vi "Instrument Setup.vi"(3 "Configured Inst":T1[](array[typedef])=[{"Public"={"Column Name"=["Timestamp"], "Trace Color"=[13802409]}, "Private"={"Path"=path "", "VI Refnum"=refnum, "Name"="", "# of Values"=0, "Scale Factors"=[], "Display"=[], "Offset"=[1.0]}}, {"Public"={"Column Name"=["Timestamp"], "Trace Color"=[11567897]}, "Private"={"Path"=path "", "VI Refnum"=refnum, "Name"="", "# of Values"=0, "Scale Factors"=[], "Display"=[], "Offset"=[1.0]}}, {"Public"={"Column Name"=[], "Trace Color"=[]}, "Private"={"Path"=path "", "VI Refnum"=refnum, "Name"="", "# of Values"=0, "Scale Factors"=[], "Display"=[], "Offset"=[1.0]}}] {"Private"."Offset" format="%^_3e"; "Private"."Scale Factors" format="%^_3e"}) -> (1 "Configured Inst dup":T1[](array[typedef]) {"Private"."Offset" format="%^_3e"; "Private"."Scale Factors" format="%^_3e"})   [LabVIEW 2021]
uses:
  Sub Controls/Instrument Properties.ctl
  Sub Controls/Public.ctl
  Sub Controls/Private.ctl
  Sub Controls/Instrument Ref.ctl
  Sub Controls/SystemCheckBox-resize.ctl
  <vilib>/Utility/miscctls.llb/LVBoundsTypeDef.ctl
  Sub Controls/Instrument Info.ctl
panel:
  out "Scan Indicator":string="Scanning Instruments...."
  in  "Rescan":bool
  in  "Instrument List":i32(listbox)
  in  "Delete":bool
  in  "Insert":bool
  in  "Done":bool
  in  "Configured Instruments":i32(listbox)
  # "Use the buttons or drag and drop instruments from the List to the Configured column.   Arrange configured instruments in the order to be called."
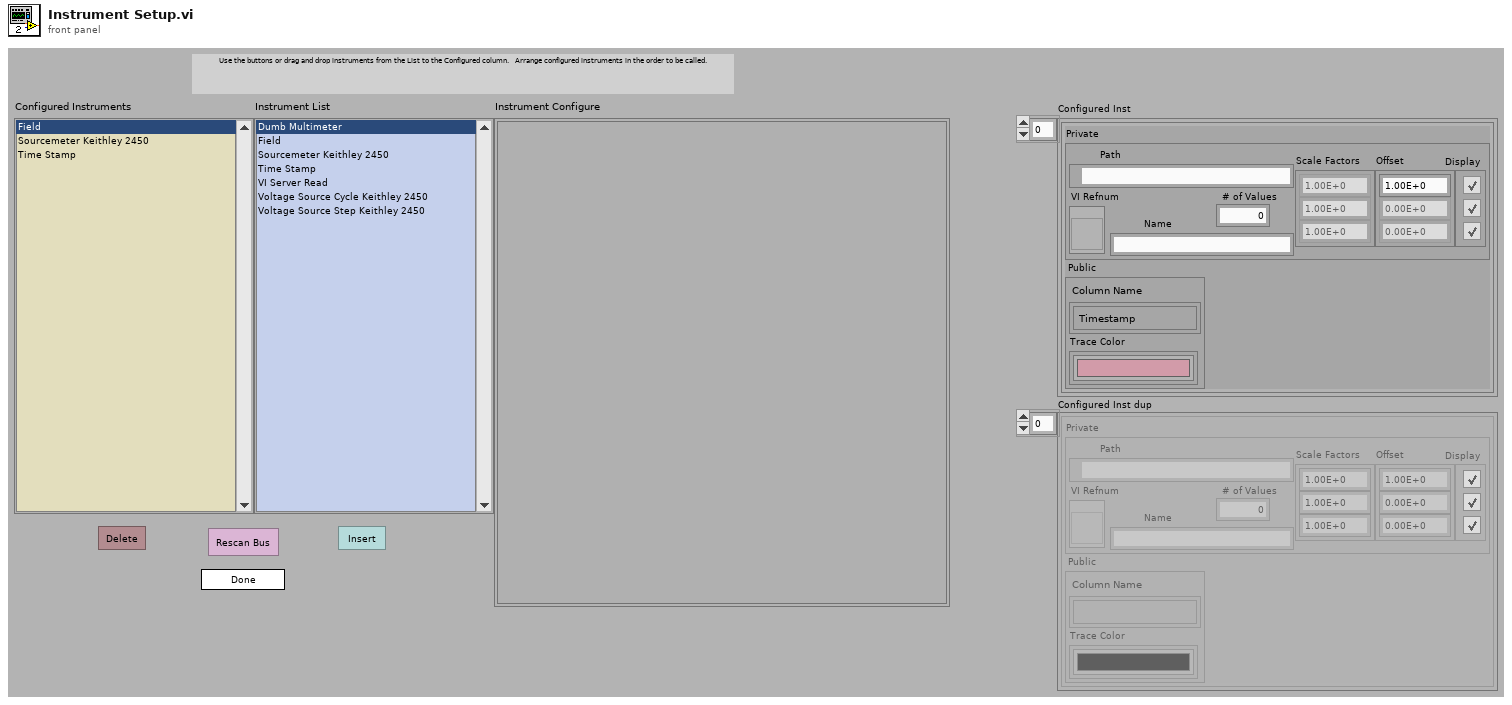
[diagram p1: front panel]
types:
  T1 = typedef "Instrument Properties.ctl" = cluster{"Public":T2, "Private":T3}
  T2 = typedef "Public.ctl" = cluster{"Column Name":string[], "Trace Color":u32[]}
  T3 = typedef "Private.ctl" = cluster{"Path":path, "VI Refnum":T4, "Name":string, "# of Values":i32, "Scale Factors":dbl[], "Display":T5[], "Offset":dbl[]}
  T4 = typedef "Instrument Ref.ctl" = refnum<vi>
  T5 = typedef "SystemCheckBox-resize.ctl" = bool
  T6 = typedef "Instrument Info.ctl" = cluster{"Name":string, "path":path}
  T7 = typedef "LVBoundsTypeDef.ctl" = cluster{"Width":u32, "Height":u32}
  T8 = enum8{"Enabled", "Disabled", "Disabled and Grayed Out"}
  T9 = typedef "Instrument IDN.ctl" = cluster{"VISA Address":string, "Status":u16, "Manufacturer":string, "Model":string, "Info":string, "Info 2":string, "Misc Data":variant}
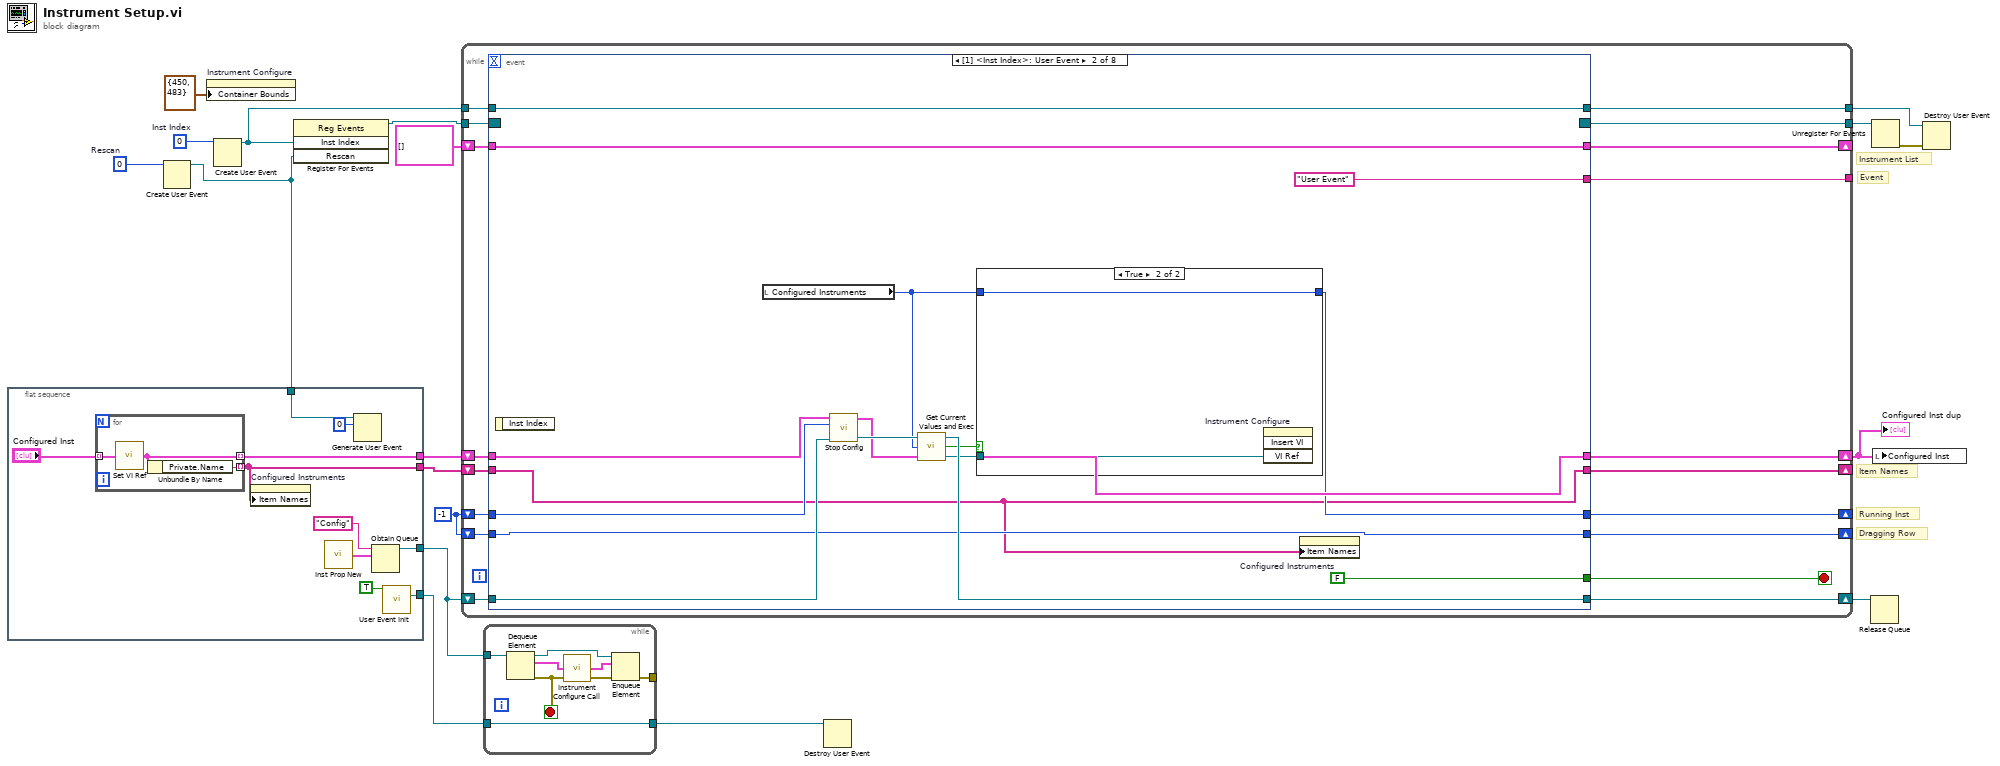
[diagram p0: block diagram]
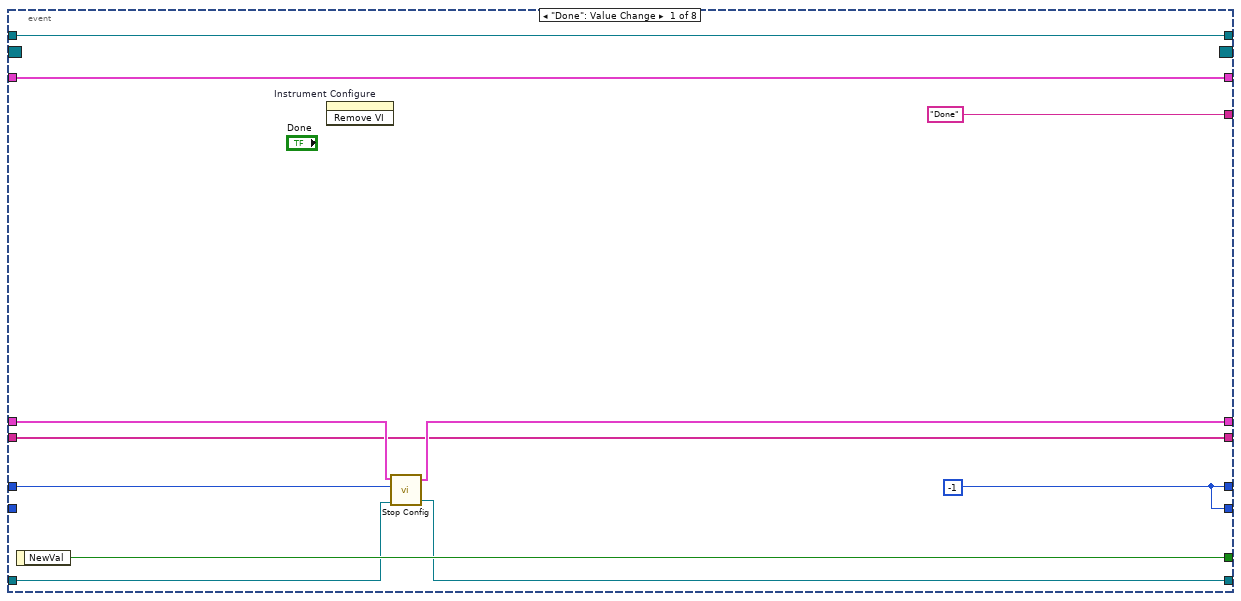
[diagram p2: hidden frame]
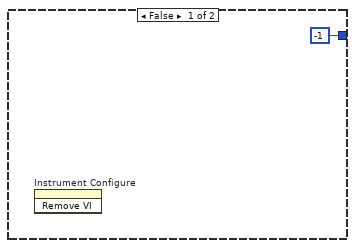
[diagram p3: hidden frame]
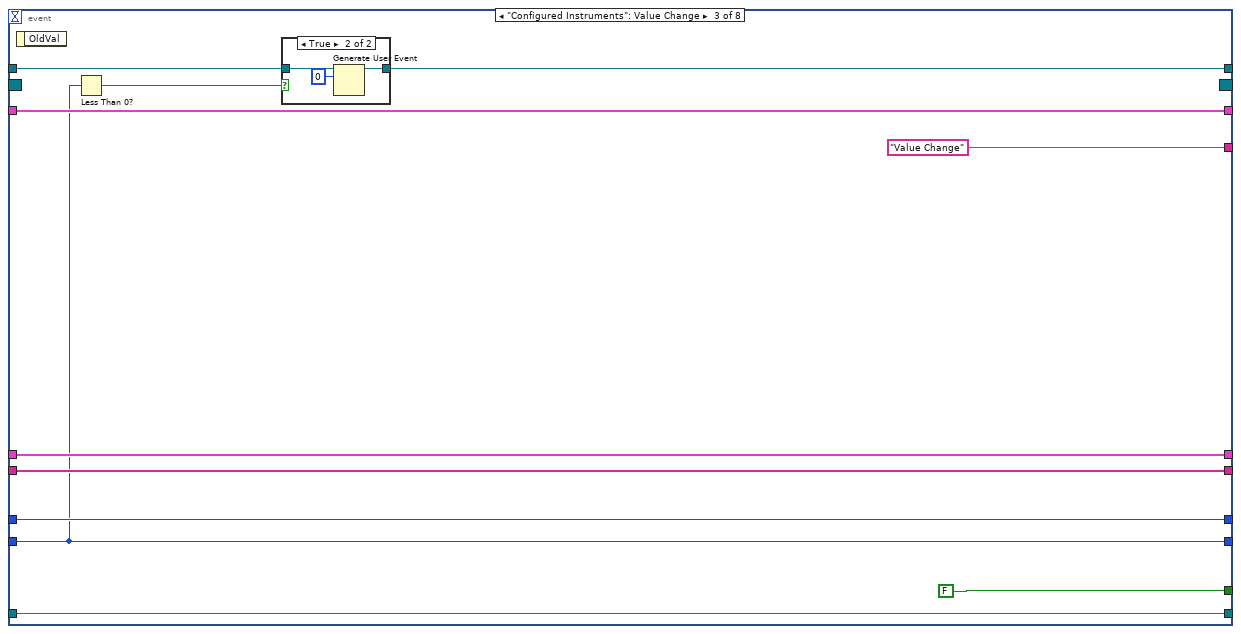
[diagram p4: hidden frame]
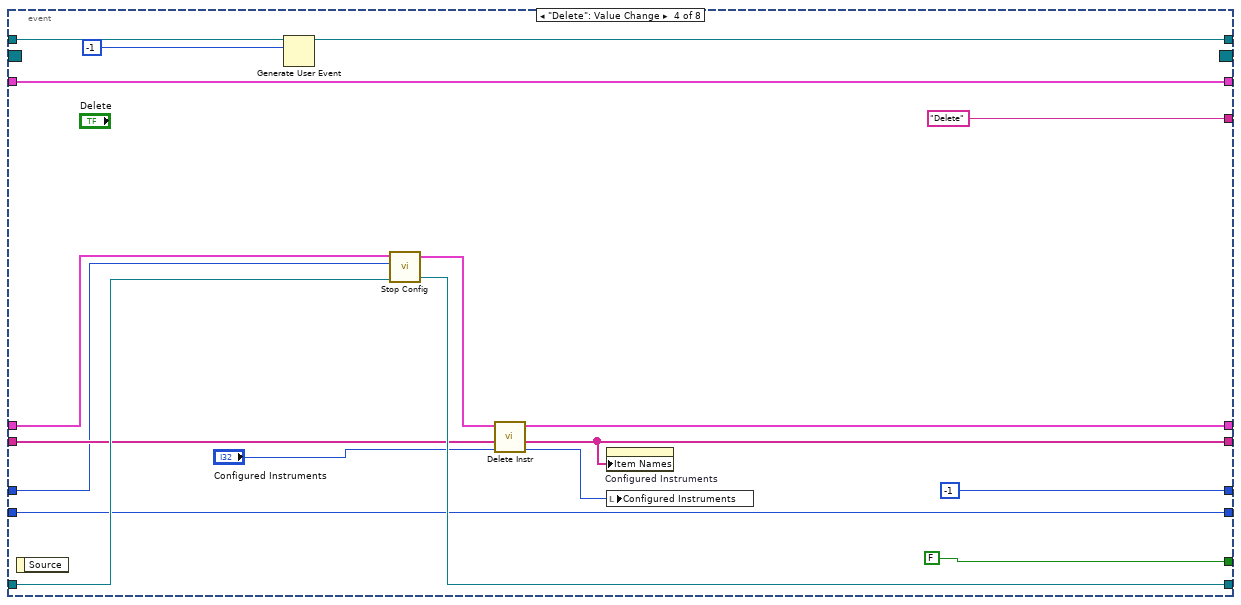
[diagram p6: hidden frame]
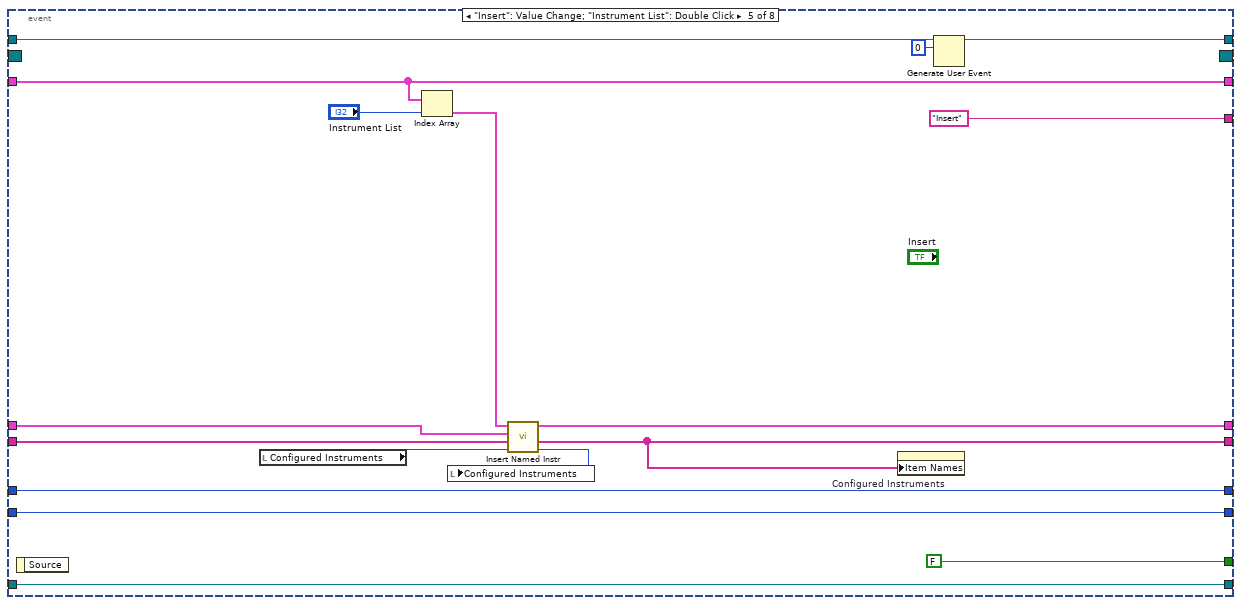
[diagram p7: hidden frame]
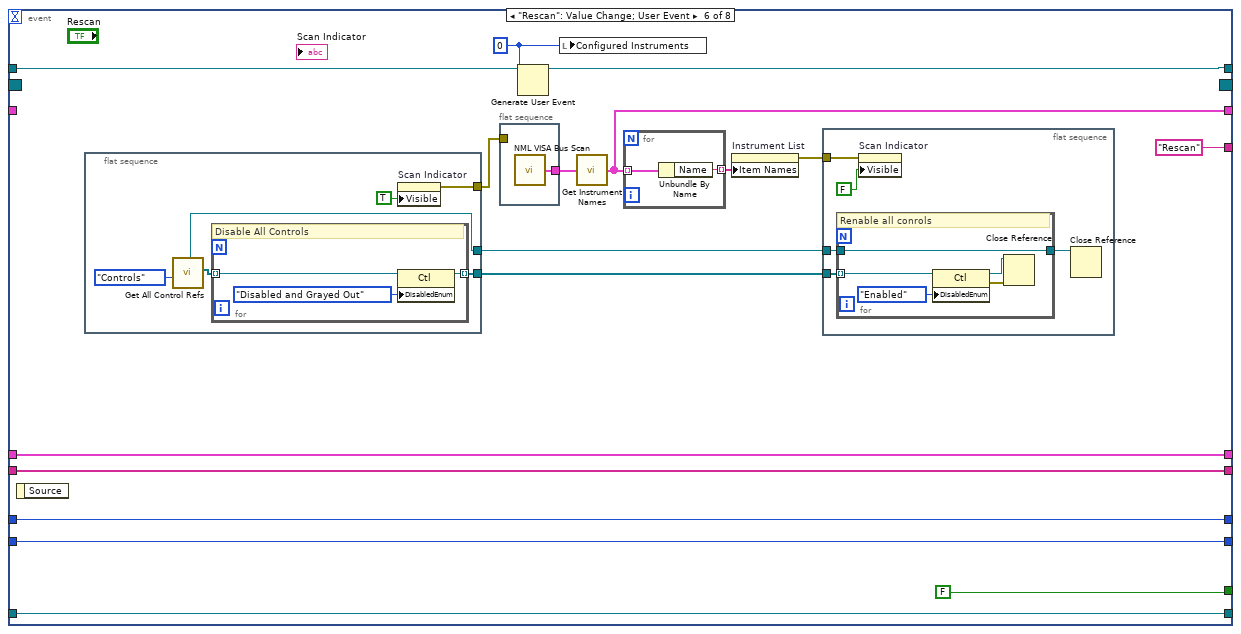
[diagram p8: hidden frame]
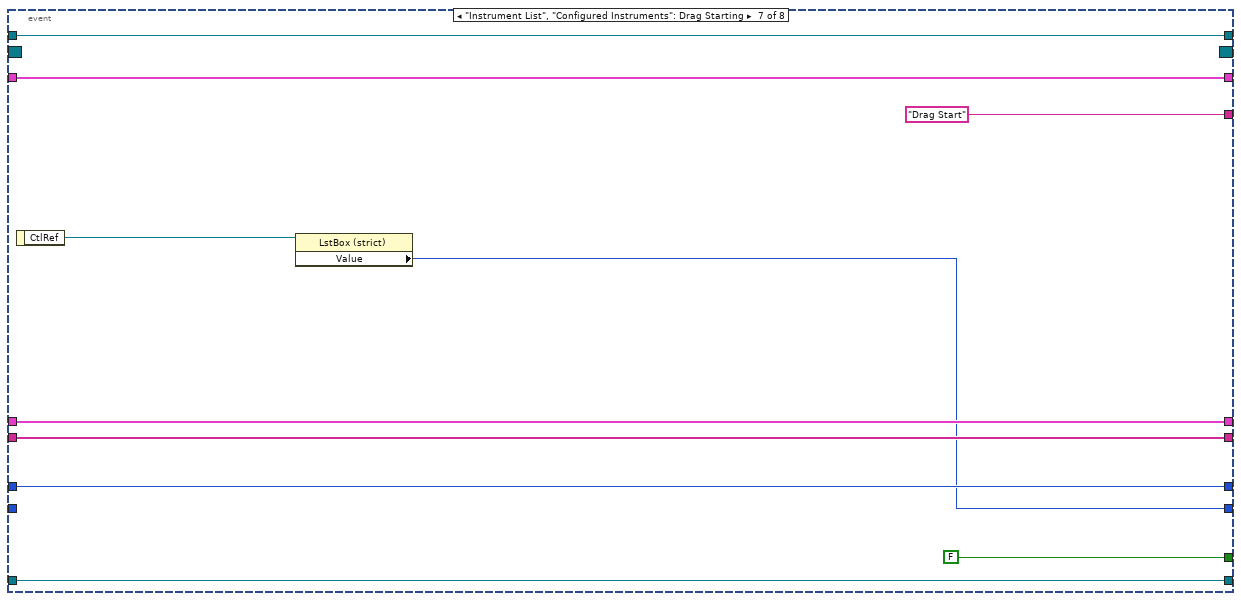
[diagram p9: hidden frame]
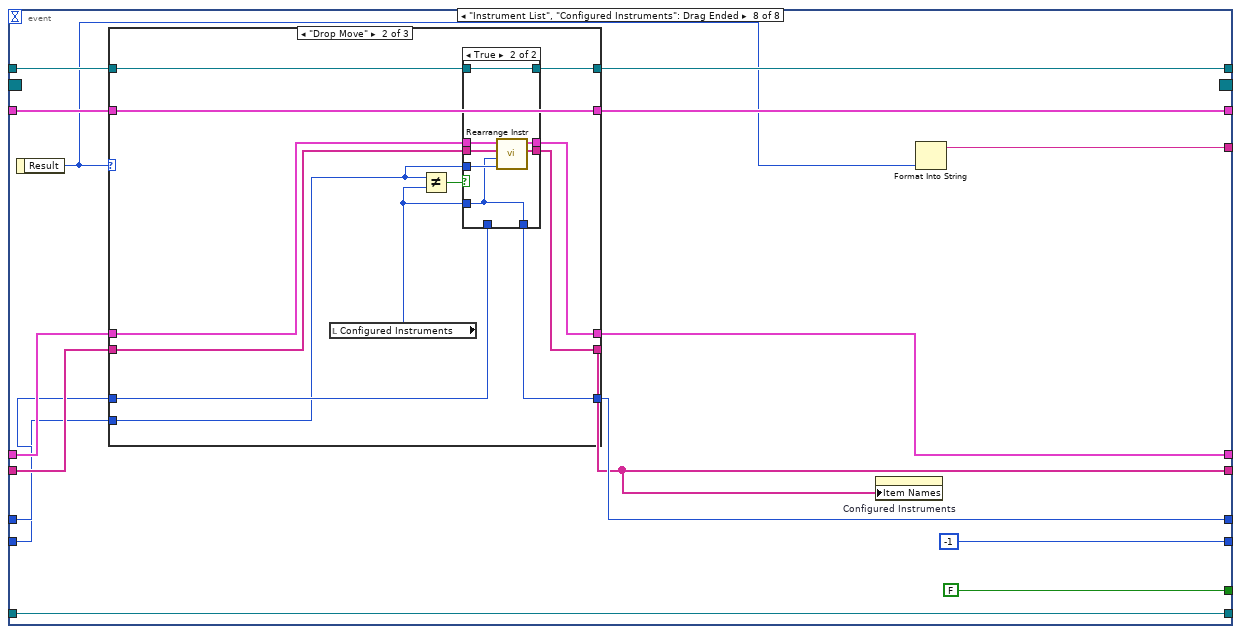
[diagram p10: hidden frame]
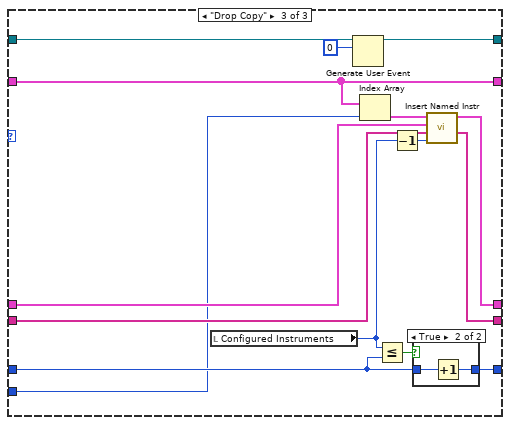
[diagram p13: hidden frame]
diagram:
  w3 = 0  # Rescan
  w6 = -1 ("SubVI Is Running")
  w4 = 0  # Inst Index
  # "Event"
  # "Dragging Row"
  # "Instrument List"
  # "Item Names"
  # "Running Inst"
  n1 = flat-sequence {
    tunnel: [w26] -> w17
    tunnel: [w21] -> w16
    tunnel: [w22] -> w15
    tunnel: [w23] -> w13
    tunnel: w1 -> [w20]
    frame #0 {
      n2 = for {
        tunnel: "Configured Inst" -> [w31] mode=indexing
        tunnel: [w29] -> w21 mode=indexing
        tunnel: [w30] -> w26 mode=indexing
        n3 = call "Set VI Ref.vi"("Instrument Prop In"=w31) -> ("Instrument Prop Out"=w30:T1)
        n4 = Unbundle By Name(w30) -> ("Private.Name"=w29:string)
      }
      n5 = property on="Configured Instruments" class="LstBox (strict)"("Item Names"=w21) -> ()  [unwired: 2 in, 2 out]
      n6 = call "Inst Prop New.vi"() -> ("Instrument Prop Out"=w25:T1)
      n7 = Generate User Event(user event=w20, event data cluster=0 ("event data")) -> ()  [unwired: 2 in, 2 out]
      n8 = Obtain Queue(name (unnamed)="Config", element data type=w25) -> (queue out=w22:refnum<queue>)  [unwired: 3 in, 2 out]
      n9 = call "User Event Init.vi"("init?"=TRUE) -> ("main menu User Event"=w23:refnum<user-event>)  [unwired: 13 in, 1 out]
    }
  }
  n10 = Create User Event(user event datatype=w3) -> (user event=w1:refnum<user-event>)  [unwired: 1 in, 1 out]
  n11 = property on="Instrument Configure" class="SubPnl"("Container Bounds"=T7 {"Width"=450, "Height"=483}) -> ()  [unwired: 2 in, 2 out]
  n12 = Create User Event(user event datatype=w4) -> (user event=w7:refnum<user-event>)  [unwired: 1 in, 1 out]
  n13 = register-events(w7, w1) -> (reference out=w11:refnum<event-registration>)  [unwired: 2 in, 1 out]
  n14 = while {
    shift-right: [w46] -> w18
    shift-left: w17 -> [w48]
    shift-right: [w37] -> _
    shift-left: w16 -> [w47]
    shift-right: [w44] -> _
    shift-left: T6[] [] ("Names") -> [w45]
    shift-right: [w40] -> w14
    shift-left: w15 -> [w43]
    tunnel: w11 -> [w42]
    tunnel: [w41] -> w9
    tunnel: w7 -> [w39]
    tunnel: [w38] -> w8
    shift-right: [w35] -> _
    shift-left: w6 -> [w36]
    tunnel: [w34] -> _
    shift-right: [w33] -> _
    shift-left: w6 -> [w32]
    stop <- w49 stop-if-true
    n15 = event shown="[1] <Inst Index>: User Event" {
      selector: w42 -> [_ _ _ _ _ _ _ _]
      dyn-events: [_ _ _ _ _ _ _ _] -> w41
      timeout: _ -> [_ _ _ _ _ _ _ _]
      tunnel: [w60 FALSE ("Done") FALSE ("Done") FALSE ("Done") FALSE ("Done") FALSE ("Done") FALSE ("Done") FALSE ("Done")] -> w49
      tunnel: w48 -> [w58 w68 w90 w104 w121 w145 w174 w189]
      tunnel: [w57 w67 w90 w99 w125 w145 w174 w190] -> w46
      tunnel: w47 -> [w53 w61 w84 w101 w118 w143 w173 w188]
      tunnel: w45 -> [w59 w75 w88 w111 w126 _ w175 w192]
      tunnel: [w59 w75 w88 w111 w126 w142 w175 w191] -> w44
      tunnel: w43 -> [w56 w70 w87 w105 w122 w144 w177 w194]
      tunnel: [w55 w76 w87 w106 w122 w144 w177 w194] -> w40
      tunnel: w39 -> [w54 w74 w85 w109 w123 w134 w176 w186]
      tunnel: [w54 w74 w86 w110 w124 w131 w176 w187] -> w38
      tunnel: [w53 w61 w84 w100 w116 w143 w173 w183] -> w37
      tunnel: w36 -> [w50 w62 w83 w95 w115 w140 w171 w185]
      tunnel: [w51 w65 w83 -1 ("SubVI Is Running") w115 w140 w171 w184] -> w35
      tunnel: ["Done" "User Event" "Value Change" "Delete" "Insert" "Rescan" "Drag Start" w182] -> w34
      tunnel: [w51 w63 w80 w96 w113 w138 w169 -1 ("SubVI Is Running")] -> w33
      tunnel: w32 -> [_ w63 w80 w96 w113 w138 _ w179]
      event "Done": Value Change {
        w51 = -1 ("SubVI Is Running")
        n16 = event-data() -> ("NewVal"=w60:bool)  [unwired: 1 in]
        n17 = invoke on="Instrument Configure" class="SubPnl" method="Remove VI"() -> ()  [unwired: 3 in, 3 out]
        n18 = call "Stop Config.vi"("queue in"=w56, "SubVI Is Running"=w50, "Array"=w58) -> ("queue out"=w55:refnum<queue>, "Array Out"=w57:T1[])  [unwired: 2 in]
      }
      event User Event {
        n19 = event-data() -> ()  [unwired: 1 in, 1 out]
        n20 = local read "Configured Instruments"() -> (w66:i32)
        n21 = call "Stop Config.vi"("queue in"=w70, "SubVI Is Running"=w62, "Array"=w68) -> ("queue out"=w69:refnum<queue>, "Array Out"=w67:T1[])  [unwired: 2 in]
        n22 = call "Get Current Values and Exec.vi"("Instrument Array"=w67, "Instrument List"=w66, "queue in"=w69) -> ("VI Ref"=w72:T4, "Valid"=w71:bool, "queue out"=w76:refnum<queue>)
        n23 = case shown="True" w71 {
          tunnel: w72 -> [_ w79]
          tunnel: w66 -> [_ w78]
          tunnel: [-1 ("Configured Instruments") w78] -> w65
          frame False {
            n24 = invoke on="Instrument Configure" class="SubPanel" method="Remove VI"() -> ()  [unwired: 3 in, 3 out]
          }
          frame True {
            n25 = invoke on="Instrument Configure" class="SubPanel" method="Insert VI"("VI Ref"=w79) -> ()  [unwired: 3 in, 4 out]
          }
        }
        n26 = property on="Configured Instruments" class="LstBox (strict)"("Item Names"=w61) -> ()  [unwired: 2 in, 2 out]
      }
      event "Configured Instruments": Value Change {
        n27 = event-data() -> ()  [unwired: 1 in, 1 out]
        n28 = Less Than 0?(x=w80) -> (x < 0?=w81:bool)
        n29 = case shown="True" w81 {
          tunnel: [w91 w94] -> w86
          tunnel: w85 -> [w91 w93]
          frame False {
          }
          frame True {
            n30 = Generate User Event(user event=w93, event data cluster=0 ("event data")) -> (user event out=w94:refnum<user-event>)  [unwired: 2 in, 1 out]
          }
        }
      }
      event "Delete": Value Change {
        n31 = event-data() -> ()  [unwired: 1 in, 1 out]
        n32 = Generate User Event(user event=w109, event data cluster=-1 ("event data")) -> (user event out=w110:refnum<user-event>)  [unwired: 2 in, 1 out]
        n33 = call "Stop Config.vi"("queue in"=w105, "SubVI Is Running"=w95, "Array"=w104) -> ("queue out"=w106:refnum<queue>, "Array Out"=w103:T1[])  [unwired: 2 in]
        n34 = call "Delete Instr.vi"("Instrument List"="Configured Instruments", "Item Names"=w101, "Setup"=w103) -> ("Instrument List Out"=w108:i32, "Item Names Out"=w100:string[], "Setup Out"=w99:T1[])  [unwired: 2 in]
        n35 = property on="Configured Instruments" class="LstBox (strict)"("Item Names"=w100) -> ()  [unwired: 2 in, 2 out]
        n36 = local write "Configured Instruments"(w108) -> ()
      }
      event "Insert": Value Change; "Instrument List": Double Click {
        n37 = event-data() -> ()  [unwired: 1 in, 1 out]
        n38 = local read "Configured Instruments"() -> (w119:i32)
        n39 = Index Array(array=w126, index="Instrument List") -> (element=w127:T6)
        n40 = call "Insert Named Instr.vi"("new instrument"=w127, "Setup"=w121, "Configured Names"=w118, "Instrument List"=w119) -> ("dup Setup"=w125:T1[], "Item Names"=w116:string[], "Instrument List Out"=w120:i32)  [unwired: 2 in]
        n41 = local write "Configured Instruments"(w120) -> ()
        n42 = property on="Configured Instruments" class="LstBox (strict)"("Item Names"=w116) -> ()  [unwired: 2 in, 2 out]
        n43 = Generate User Event(user event=w123, event data cluster=0 ("event data")) -> (user event out=w124:refnum<user-event>)  [unwired: 2 in, 1 out]
      }
      event "Rescan": Value Change; User Event {
        w135 = 0 ("Instrument List")
        n44 = event-data() -> ()  [unwired: 1 in, 1 out]
        n45 = flat-sequence {
          tunnel: [w151] -> w137
          tunnel: [w148] -> w133
          tunnel: [w147] -> w132
          frame #0 {
            # "Disable Controls"
            n46 = call "Get All Control Refs.vi"("Type"=enum16{"Both", "Controls", "Indicators"}."Controls" ("Enum")) -> ("VI Refnum"=w148:refnum<vi>, "All Controls"=w150:refnum<vi>[])  [unwired: 5 in, 1 out]
            n47 = for {
              tunnel: w150 -> [w155] mode=indexing
              tunnel: [w153] -> w147 mode=indexing
              # "Disable All Controls"
              n48 = property class="Ctl"(reference=w155, "DisabledEnum"=T8."Disabled and Grayed Out" ("Disabled")) -> (reference out=w153:refnum<vi>)  [unwired: 1 in, 1 out]
            }
            n49 = property on="Scan Indicator" class="Str"("Visible"=TRUE) -> (error out=w151:errorcluster)  [unwired: 2 in, 1 out]
          }
        }
        n50 = flat-sequence {
          tunnel: [w166] -> w130
          tunnel: w137 -> [_]
          frame #0 {
            n51 = call "NML VISA Bus Scan.vi"() -> ("Instrument List"=w166:T9[])  [unwired: 1 in]
          }
        }
        n52 = Generate User Event(user event=w134, event data cluster=w135) -> (user event out=w131:refnum<user-event>)  [unwired: 2 in, 1 out]
        n53 = local write "Configured Instruments"(w135) -> ()
        n54 = call "Get Instrument Names.vi"("Instrument List"=w130) -> ("Names"=w142:T6[])
        n55 = for {
          tunnel: w142 -> [w168] mode=indexing
          tunnel: [w167] -> w141 mode=indexing
          n56 = Unbundle By Name(w168) -> ("Name"=w167:string)
        }
        n57 = property on="Instrument List" class="LstBox (strict)"("Item Names"=w141) -> (error out=w136:errorcluster)  [unwired: 2 in, 1 out]
        n58 = flat-sequence {
          tunnel: w136 -> [w159]
          tunnel: w133 -> [w157]
          tunnel: w132 -> [w156]
          frame #0 {
            # "Re-en"
            n59 = for {
              tunnel: w156 -> [w165] mode=indexing
              tunnel: w157 -> [w161]
              tunnel: [w161] -> w158
              # "Renable all conrols"
              n60 = property class="Ctl"(reference=w165, "DisabledEnum"=T8."Enabled" ("Disabled")) -> (reference out=w162:refnum<vi>, error out=w163:errorcluster)  [unwired: 1 in]
              n61 = Close Reference(reference=w162, error in (no error)=w163) -> ()  [unwired: 1 out]
            }
            n62 = property on="Scan Indicator" class="Str"(error in=w159, "Visible"=FALSE) -> ()  [unwired: 1 in, 2 out]
            n63 = Close Reference(reference=w158) -> ()  [unwired: 1 in, 1 out]
          }
        }
      }
      event "Instrument List", "Configured Instruments": Drag Starting {
        n64 = event-data() -> ("CtlRef"=w178:refnum<vi>)  [unwired: 1 in]
        n65 = property class="LstBox (strict)"(reference=w178) -> ("Value"=w169:i32)  [unwired: 1 in, 2 out]
      }
      event "Instrument List", "Configured Instruments": Drag Ended {
        n66 = event-data() -> ("Result"=w181:enum16{"Drop Cancel", "Drop Move", "Drop Copy"})  [unwired: 1 in]
        n67 = case shown="\"Drop Move\"" w181 {
          tunnel: w192 -> [w199 w205 w236]
          tunnel: [w199 w205 w236] -> w191
          tunnel: [w198 w209 w235] -> w190
          tunnel: w189 -> [w198 w210 w234]
          tunnel: [w197 w208 w233] -> w183
          tunnel: w188 -> [w197 w211 w232]
          tunnel: [w196 w207 w231] -> w187
          tunnel: w186 -> [w196 w206 w230]
          tunnel: [w195 w202 w225] -> w184
          tunnel: w185 -> [w195 w201 w224]
          tunnel: w179 -> [_ w200 w223]
          frame "Drop Cancel", Default {
          }
          frame "Drop Move" {
            n68 = local read "Configured Instruments"() -> (w203:i32)
            n69 = Not Equal?(x=w200, y=w203) -> (x != y?=w204:bool)
            n70 = case shown="True" w204 {
              tunnel: w211 -> [w213 w222]
              tunnel: w210 -> [w214 w221]
              tunnel: [w214 w220] -> w209
              tunnel: [w213 w219] -> w208
              tunnel: [w215 w218] -> w207
              tunnel: w206 -> [w215 w218]
              tunnel: w200 -> [_ w217]
              tunnel: w203 -> [_ w216]
              tunnel: [w212 w216] -> w202
              tunnel: w201 -> [w212 _]
              frame False {
              }
              frame True {
                n71 = call "Rearrange Instr.vi"("Item to Move"=w217, "Insert At"=w216, "Configured Names"=w222, "Setup In"=w221) -> ("Item Names"=w219:string[], "Setup Out"=w220:T1[])  [unwired: 3 in, 1 out]
              }
            }
          }
          frame "Drop Copy" {
            n72 = local read "Configured Instruments"() -> (w229:i32)
            n73 = Generate User Event(user event=w230, event data cluster=0 ("event data")) -> (user event out=w231:refnum<user-event>)  [unwired: 2 in, 1 out]
            n74 = Index Array(array=w236, index=w223) -> (element=w237:T6)
            n75 = Less Or Equal?(x=w229, y=w224) -> (x <= y?=w228:bool)
            n76 = Decrement(x=w229) -> (x-1=w226:i32)
            n77 = case shown="True" w228 {
              tunnel: w224 -> [w238 w240]
              tunnel: [w238 w239] -> w225
              frame False {
              }
              frame True {
                n78 = Increment(x=w240) -> (x+1=w239:i32)
              }
            }
            n79 = call "Insert Named Instr.vi"("new instrument"=w237, "Setup"=w234, "Configured Names"=w232, "Instrument List"=w226) -> ("dup Setup"=w235:T1[], "Item Names"=w233:string[])  [unwired: 2 in, 1 out]
          }
        }
        n80 = property on="Configured Instruments" class="LstBox (strict)"("Item Names"=w183) -> ()  [unwired: 2 in, 2 out]
        n81 = Format Into String(w181) -> (resulting string=w182:string)  [unwired: 3 in, 1 out]
      }
    }
  }
  "Configured Inst dup" <- w18
  n82 = while {
    tunnel: w15 -> [w248]
    tunnel: [w243] -> _
    tunnel: [w242] -> w12
    tunnel: w13 -> [w242]
    stop <- w247 stop-if-true
    n83 = Dequeue Element(queue=w248) -> (queue out=w241:refnum<queue>, element=w246:T1, error out=w247:errorcluster)  [unwired: 2 in, 1 out]
    n84 = call "Instrument Configure Call.vi"("error in"=w247, "Instrument Prop In"=w246) -> ("error out"=w244:errorcluster, "Instrument Prop Out"=w245:T1)  [unwired: 2 in]
    n85 = Enqueue Element(queue=w241, element=w245, error in (no error)=w244) -> (error out=w243:errorcluster)  [unwired: 1 in, 2 out]
  }
  n86 = Destroy User Event(user event=w12) -> ()  [unwired: 1 in, 1 out]
  n87 = Release Queue(queue=w14) -> ()  [unwired: 2 in, 3 out]
  n88 = Unregister For Events(event registration refnum=w9) -> (error out=w10:errorcluster)  [unwired: 1 in]
  n89 = local write "Configured Inst"(w18) -> ()
  n90 = Destroy User Event(user event=w8, error in=w10) -> ()  [unwired: 1 out]
